vi "Verify Expected Options.vi"(0 "Expected Options":string, 5 "Reported Options":string, 11 "error in (no error)":errorcluster) -> (4 "Mismatch? (True = Mismatch)":bool, 15 "error out":errorcluster)   [LabVIEW 2018]
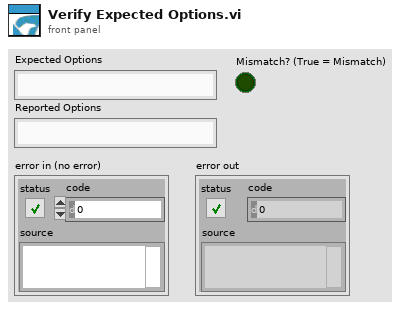
[diagram p1: front panel]
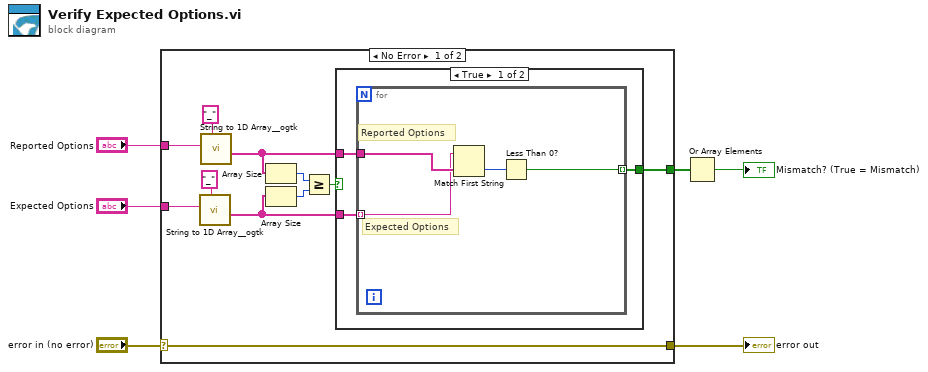
[diagram p0: block diagram]
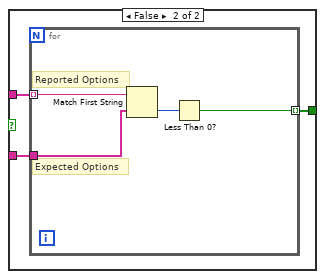
[diagram p2: hidden frame]
diagram:
  n1 = case shown="No Error" "error in (no error)" {
    selector: "error in (no error)" -> [w13 w32]
    tunnel: [w13 w32] -> w5
    tunnel: "Reported Options" -> [w17 _]
    tunnel: "Expected Options" -> [w14 _]
    tunnel: [w7 _] -> w2
    frame No Error {
      n2 = call <userlib>:"String to 1D Array__ogtk.vi"("delimiter (Tab)"="_", "string"=w14) -> ("Array of Strings"=w8:string[])  [unwired: 9 in]
      n3 = call <userlib>:"String to 1D Array__ogtk.vi"("delimiter (Tab)"="_", "string"=w17) -> ("Array of Strings"=w9:string[])  [unwired: 9 in]
      n4 = Array Size(array=w9) -> (size(s)=w12:i32)
      n5 = Array Size(array=w8) -> (size(s)=w11:i32)
      n6 = Greater Or Equal?(x=w12, y=w11) -> (x >= y?=w10:bool)
      n7 = case shown="True" w10 {
        tunnel: w9 -> [w20 w27]
        tunnel: w8 -> [w19 w26]
        tunnel: [w18 w25] -> w7
        frame True {
          n8 = for {
            tunnel: w20 -> [w24]
            tunnel: w19 -> [w23] mode=indexing
            tunnel: [w21] -> w18 mode=indexing
            # "Reported Options"
            # "Expected Options"
            n9 = Match First String(2:w24, 3:w23) -> (0:w22:i32)  [unwired: 1 out]
            n10 = Less Than 0?(x=w22) -> (x < 0?=w21:bool)
          }
        }
        frame False {
          n11 = for {
            tunnel: w27 -> [w28] mode=indexing
            tunnel: w26 -> [w29]
            tunnel: [w30] -> w25 mode=indexing
            # "Reported Options"
            # "Expected Options"
            n12 = Match First String(2:w29, 3:w28) -> (0:w31:i32)  [unwired: 1 out]
            n13 = Less Than 0?(x=w31) -> (x < 0?=w30:bool)
          }
        }
      }
    }
    frame Error {
    }
  }
  "error out" <- w5
  n14 = Or Array Elements(Boolean array=w2) -> (logical OR=→"Mismatch? (True = Mismatch)":bool)
